vi "FpgaSession_SET.vi"(8 "error in":errorcluster, 10 "fpga session in":refnum<k20>, 11 "lia host in":refnum<class "LIA Host Interface FPGA.lvclass">) -> (0 "error out":errorcluster, 3 "lia host out":refnum<class "LIA Host Interface FPGA.lvclass">)   [LabVIEW 2018, in "LIA Host Interface FPGA.lvclass"]
uses:
  LIA Host Interface FPGA.lvclass
  LIA Host Interface FPGA.lvclass/LIA Host Interface FPGA.ctl
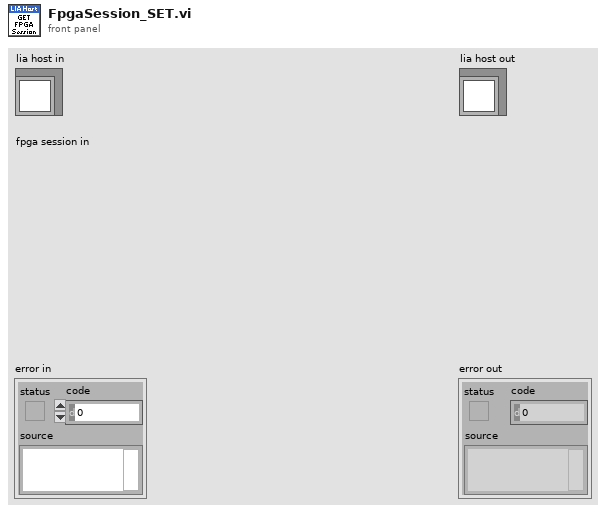
[diagram p1: front panel]
types:
  T1 = typedef "LIA Host Interface Desktop.lvclass/session data.ctl" = cluster{"fpga session":refnum<k20>, "record length":u32[]}
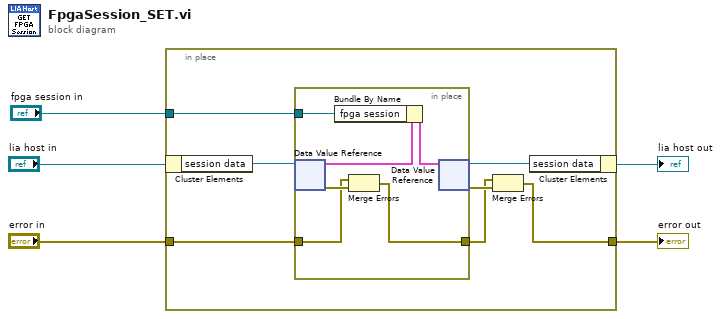
[diagram p0: block diagram]
diagram:
  n1 = in-place {
    in-place-border: "error in" -> [w10]
    in-place-border: [w7] -> w2
    in-place-border: "fpga session in" -> [w6]
    n2 = in-place-cluster #1("lia host in") -> ("session data"=w12:refnum<data-value>)
    n3 = in-place {
      in-place-border: w10 -> [w16]
      in-place-border: [w15] -> w8
      in-place-border: w6 -> [w13]
      n4 = in-place-dvr #2(w12) -> (w18:T1, w17:errorcluster)
      n5 = Bundle By Name(cluster=w18, "fpga session"=w13) -> (w14:T1)
      n6 = Merge Errors(w16, w17) -> (w15:errorcluster)
      n7 = in-place-dvr #2(w14) -> (w11:refnum<data-value>, w9:errorcluster)
    }
    n8 = Merge Errors(w8, w9) -> (w7:errorcluster)
    n9 = in-place-cluster #1("session data"=w11) -> (→"lia host out":refnum<class "LIA Host Interface FPGA.lvclass">)
  }
  "error out" <- w2
